vi "Create Sequence Main.vi"(0 "project path":path, 5 "measurement name":string, 11 "error in":errorcluster) -> (15 "error out":errorcluster)   [LabVIEW 2021, in "Create Sequence.lvlib"]
uses:
  Create Sequence.lvlib
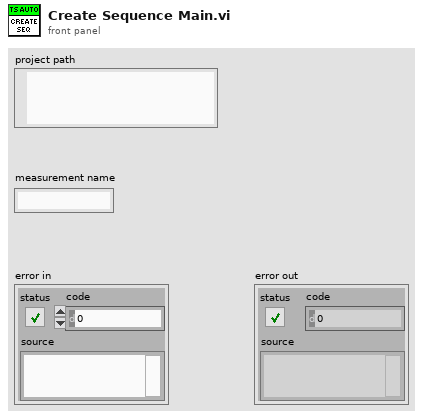
[diagram p1: front panel]
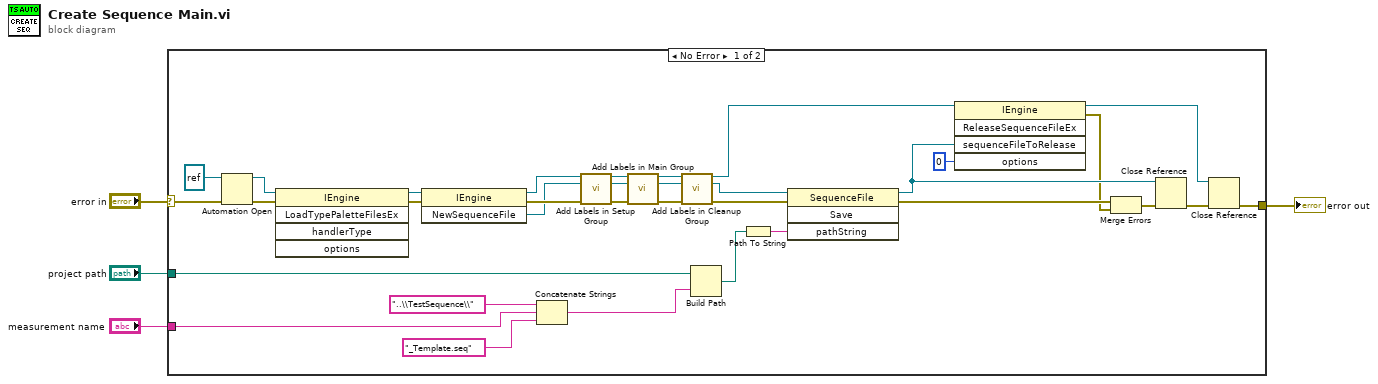
[diagram p0: block diagram]
diagram:
  n1 = case shown="No Error" "error in" {
    selector: "error in" -> [w21 w38]
    tunnel: [w33 w38] -> w1
    tunnel: "measurement name" -> [w12 _]
    tunnel: "project path" -> [w10 _]
    frame No Error {
      n2 = Automation Open(error in (no error)=w21, Automation Refnum=refnum<k7> refnum) -> (Automation Refnum=w25:refnum<k7>, error out=w29:errorcluster)  [unwired: 2 in]
      n3 = invoke class="IEngine" method="LoadTypePaletteFilesEx"(reference=w25, error in=w29) -> (reference out=w30:refnum<k7>, error out=w28:errorcluster)  [unwired: 3 in, 3 out]
      n4 = invoke class="IEngine" method="NewSequenceFile"(reference=w30, error in=w28) -> (reference out=w32:refnum<k7>, error out=w31:errorcluster, "NewSequenceFile"=w26:refnum<k7>)  [unwired: 1 in]
      n5 = Concatenate Strings("..\\TestSequence\\" ("string"), w12, "_Template.seq" ("string")) -> (w14:string)
      n6 = call "Add Labels in Setup Group.vi"("engine in"=w32, "sequence file in"=w26, "error in"=w31) -> ("engine out"=w19:refnum<k7>, "sequence file out"=w17:refnum<k7>, "error out"=w15:errorcluster)  [unwired: 10 in]
      n7 = call "Add Labels in Main Group.vi"("engine in"=w19, "sequence file in"=w17, "error in"=w15) -> ("engine out"=w20:refnum<k7>, "sequence file out"=w18:refnum<k7>, "error out"=w16:errorcluster)  [unwired: 10 in]
      n8 = call "Add Labels in Cleanup Group.vi"("engine in"=w20, "sequence file in"=w18, "error in"=w16) -> ("engine out"=w24:refnum<k7>, "sequence file out"=w23:refnum<k7>, "error out"=w22:errorcluster)  [unwired: 10 in]
      n9 = Build Path(base path=w10, name or relative path=w14) -> (appended path=w8:path)
      n10 = Path To String(path=w8) -> (string=w7:string)
      n11 = invoke class="SequenceFile" method="Save"(reference=w23, error in=w22, "pathString"=w7) -> (reference out=w35:refnum<k7>, error out=w6:errorcluster)  [unwired: 1 in, 2 out]
      n12 = invoke class="IEngine" method="ReleaseSequenceFileEx"(reference=w24, "sequenceFileToRelease"=w35, "options"=0) -> (reference out=w36:refnum<k7>, error out=w5:errorcluster)  [unwired: 2 in, 3 out]
      n13 = Merge Errors(w6, w5) -> (w34:errorcluster)
      n14 = Close Reference(reference=w35, error in (no error)=w34) -> (error out=w37:errorcluster)
      n15 = Close Reference(reference=w36, error in (no error)=w37) -> (error out=w33:errorcluster)
    }
    frame Error {
    }
  }
  "error out" <- w1
